vi "Test-Operator-Elevator.vi"() -> ()   [LabVIEW 2014, in "Comp Operator.lvlib"]
uses:
  Comp Operator.lvlib
  Robot Actor Framework/Trace/Trace Controller Class/Config.ctl
  Comp Motors with Encoders/Comp Motors with Encoders Class/Motor Controller Config.ctl
  Robot/Motor with Encoders/Motors with Encoders Class/Motors with Encoders Config.ctl
  Comp Motors with Encoders/Comp Motors with Encoders Class/Encoder Config.ctl
  Robot/Forward Drive/Forward Drive Class/Forward Drive Config.ctl
  Robot/Motor with Encoders/Motors with Encoders Class/Motors with Encoders.lvclass
  Comp Drive/Comp Driver Class/Comp Driver Tuning.ctl
  Robot/Driver/Driver Class/Driver Config.ctl
  Robot/Joystick/Joystick Class/Joystick.lvclass
  <vilib>/ActorFramework/Message Enqueuer/Message Enqueuer.lvclass
  Comp Xbox One Controller/Comp XBox One Controller Class/Comp X1 Config.ctl
  <vilib>/Rock Robotics/WPI/Joystick/WPI_JoystickDeviceEnum.ctl
  Robot/Joystick/Joystick Class/Axis State.ctl
  Robot/Joystick/Joystick Class/Button State.ctl
  Comp Trace Controller/Comp Trace Controller Class/Comp Trace Controller.lvclass
  Comp Pressure/Comp Pressure Class/Comp Pressure.lvclass
  Robot/Forward Drive/Forward Drive Class/Forward Drive.lvclass
  Comp Motors with Encoders/Comp Motors with Encoders Class/Comp Motors with Encoders.lvclass
  Comp Drive/Comp Driver Class/Comp Driver.lvclass
  Comp Xbox One Controller/Comp XBox One Controller Class/Comp XBox One Controller.lvclass
  Comp Xbox One Controller/Comp XBox One Controller Class/Comp XBox One Controller.lvclass/Comp XBox One Controller.ctl
  <vilib>/Rock Robotics/WPI/DriverStation/WPI_DriverStationRobotMode2.ctl
  Robot/Joystick/Joystick Class/Joystick State.ctl
  Robot/Driver/Driver Messages/Drive Forward Drive Msg/Drive Forward Drive Msg.lvclass/Drive Forward Drive Msg.ctl
  <vilib>/ActorFramework/Message Enqueuer/Message Enqueuer.lvclass/Message Enqueuer.ctl
  <vilib>/ActorFramework/Message Enqueuer/Enqueue.vi
  <vilib>/ActorFramework/Message Priority Queue/Priority Enqueue.vi
  Robot/Driver/Driver Messages/Drive Forward Drive Msg/Drive Forward Drive Msg.lvclass
  <vilib>/ActorFramework/Stop Msg/Stop Msg.lvclass
  <vilib>/ActorFramework/Actor/Actor.lvclass
  Robot Actor Framework/Trace/Trace Controller Class/Trace Controller.lvclass
  Robot/Driver/Driver Class/Driver.lvclass
panel:
  in  "Left Back":T1
  in  "Left Right":T1
  in  "Driver - X1 Config":T3={"Joystick USB"=enum."USB 0", "Deadband"=0.05}
  in  "Driver Config":T5={"Joystick"=refnum, "Forward Drive"=refnum, "Sideways Drive"=refnum, "Percent Forward"=1.0, "Percent Sideways"=1.0}
  in  "Comp Driver Tuning":T6={"Control Update Throttle"=75}
  in  "Test Loop":u32=50
  in  "Right Encoder Config":T7={"P"=1.0, "D"=0.0, "F"=0.01, "I"=0.01, "Reverse Feedback Sensor"=TRUE, "Encoder Codes Per Rev"=256}
  in  "Right Slaves":T8[](array[typedef])=[{"Device Number"=5, "Invert Motor"=FALSE}]
  in  "Right Master":T8={"Device Number"=4, "Invert Motor"=TRUE}
  in  "Forward Drive Config":T9={"Left Motors with Encoders"=refnum, "Right Motors with Encoders"=refnum, "Encoder Control"=TRUE}
  in  "Left Encoder Config":T7={"P"=1.0, "D"=0.0, "F"=0.01, "I"=0.01, "Reverse Feedback Sensor"=TRUE, "Encoder Codes Per Rev"=256}
  out "Enable Tele":bool caption="Enabled Teleop"
  in  "Stop Test Loop 1":bool=TRUE
  in  "Finish Test":bool=TRUE
  in  "Start Test":bool=TRUE
  in  "Motors with Encoder Config":T10={"Counts  Per Revolution"=256, "Invert Encoder Direction"=FALSE, "Diameter of Revolution"=6.0, "Max RPM"=1900.0, "Encoder Control"=TRUE}
  in  "Left Slave Motor Controller Configs":T8[](array[typedef])=[{"Device Number"=10, "Invert Motor"=FALSE}]
  in  "left Master Motor Controller Config":T8={"Device Number"=9, "Invert Motor"=FALSE}
  in  "Config":T11={"Folder Pattern"="/media/sd%s1", "Starting Letter Position"=1, "Min Free Space (MB)"=50.0, "Max Folders to Check"=10, "Trace Level"=enum."Debug"} {"Min Free Space (MB)" format="%#_13g"}
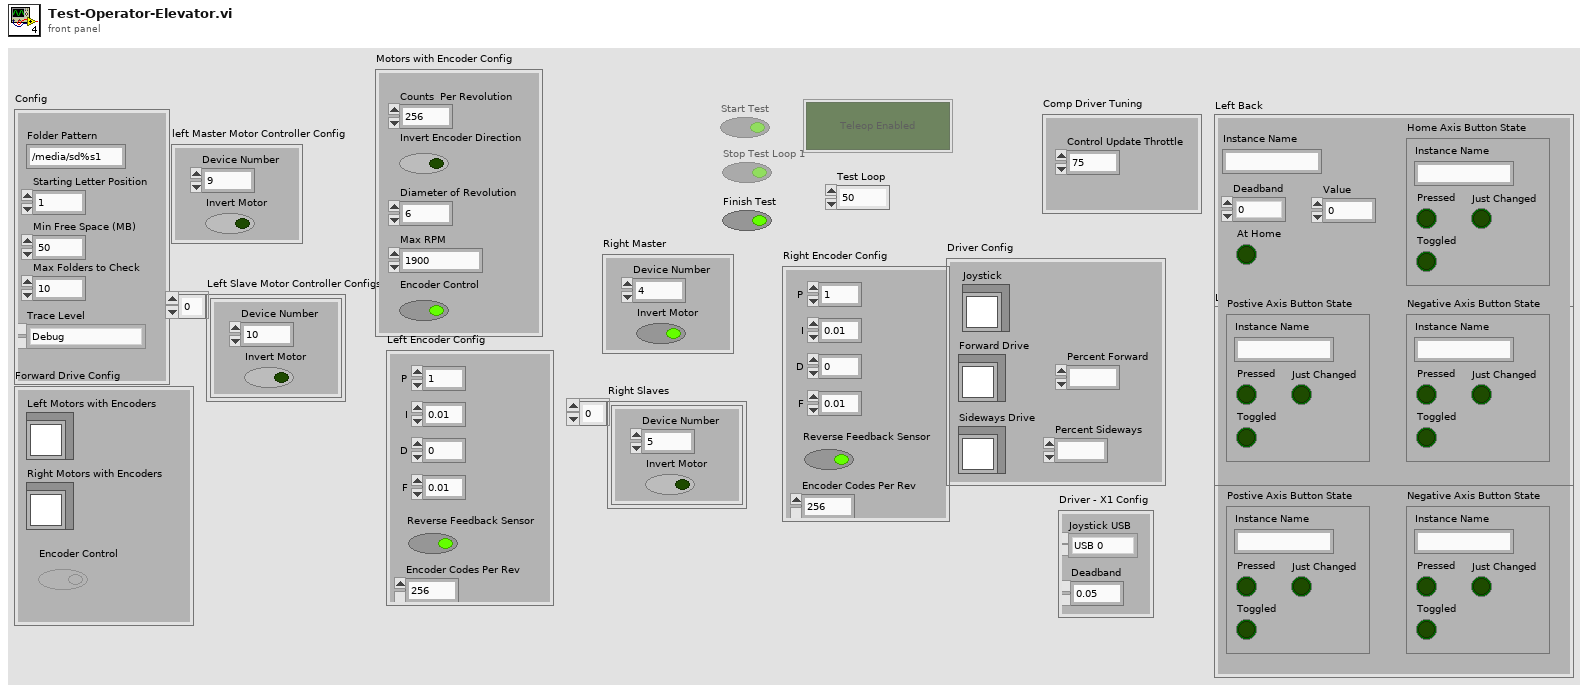
[diagram p1: front panel]
types:
  T1 = typedef "Joystick.lvlib/Joystick.lvclass/Axis State.ctl" = cluster{"Instance Name":string, "Deadband":dbl, "Value":dbl, "At Home":bool, "Postive Axis Button State":T2, "Negative Axis Button State":T2, "Home Axis Button State":T2}
  T2 = typedef "Joystick.lvlib/Joystick.lvclass/Button State.ctl" = cluster{"Pressed":bool, "Instance Name":string, "Toggled":bool, "Just Changed":bool}
  T3 = typedef "Comp XBox One Controller.lvlib/Comp XBox One Controller.lvclass/Comp X1 Config.ctl" = cluster{"Joystick USB":T4, "Deadband":dbl}
  T4 = typedef "WPI_JoystickDeviceEnum.ctl" = enum16{"USB 0", "USB 1", "USB 2", "USB 3", "USB 4", "USB 5"}
  T5 = typedef "Driver.lvlib/Driver.lvclass/Driver Config.ctl" = cluster{"Joystick":refnum<class "Joystick.lvclass">, "Forward Drive":refnum<class "Message Enqueuer.lvclass">, "Sideways Drive":refnum<class "Message Enqueuer.lvclass">, "Percent Forward":dbl, "Percent Sideways":dbl}
  T6 = typedef "Comp Driver.lvlib/Comp Driver.lvclass/Comp Driver Tuning.ctl" = cluster{"Control Update Throttle":u32}
  T7 = typedef "Comp Motors with Encoders.lvlib/Comp Motors with Encoders.lvclass/Encoder Config.ctl" = cluster{"P":dbl, "D":dbl, "F":dbl, "I":dbl, "Reverse Feedback Sensor":bool, "Encoder Codes Per Rev":u16}
  T8 = typedef "Comp Motors with Encoders.lvlib/Comp Motors with Encoders.lvclass/Motor Controller Config.ctl" = cluster{"Device Number":u8, "Invert Motor":bool}
  T9 = typedef "Forward Drive.lvlib/Forward Drive.lvclass/Forward Drive Config.ctl" = cluster{"Left Motors with Encoders":refnum<class "Motors with Encoders.lvclass">, "Right Motors with Encoders":refnum<class "Motors with Encoders.lvclass">, "Encoder Control":bool}
  T10 = typedef "Motors with Encoders.lvlib/Motors with Encoders.lvclass/Motors with Encoders Config.ctl" = cluster{"Counts  Per Revolution":u32, "Invert Encoder Direction":bool, "Diameter of Revolution":dbl, "Max RPM":dbl, "Encoder Control":bool}
  T11 = typedef "Robot Actor Framework.lvlib/Trace.lvlib/Trace Controller.lvclass/Config.ctl" = cluster{"Folder Pattern":string, "Starting Letter Position":i32, "Min Free Space (MB)":dbl, "Max Folders to Check":u32, "Trace Level":enum16{"Critical", "Error", "Warning", "Informational", "Debug"}}
  T12 = enum16{"Critical", "Error", "Warning", "Informational", "Debug"}
  T13 = enum8{"Enabled", "Disabled", "Disabled and Grayed Out"}
  T14 = typedef "WPI_DriverStationRobotMode2.ctl" = enum16{"Autonomous Disabled", "Autonomous Enabled", "Teleop Disabled", "Teleop Enabled", "Disconnected", "Finish", "Test Disabled", "Test Enabled", "Emergency Stopped"}
  T15 = typedef "Joystick.lvlib/Joystick.lvclass/Joystick State.ctl" = cluster{"Buttons":T2[], "Axis":T1[]}
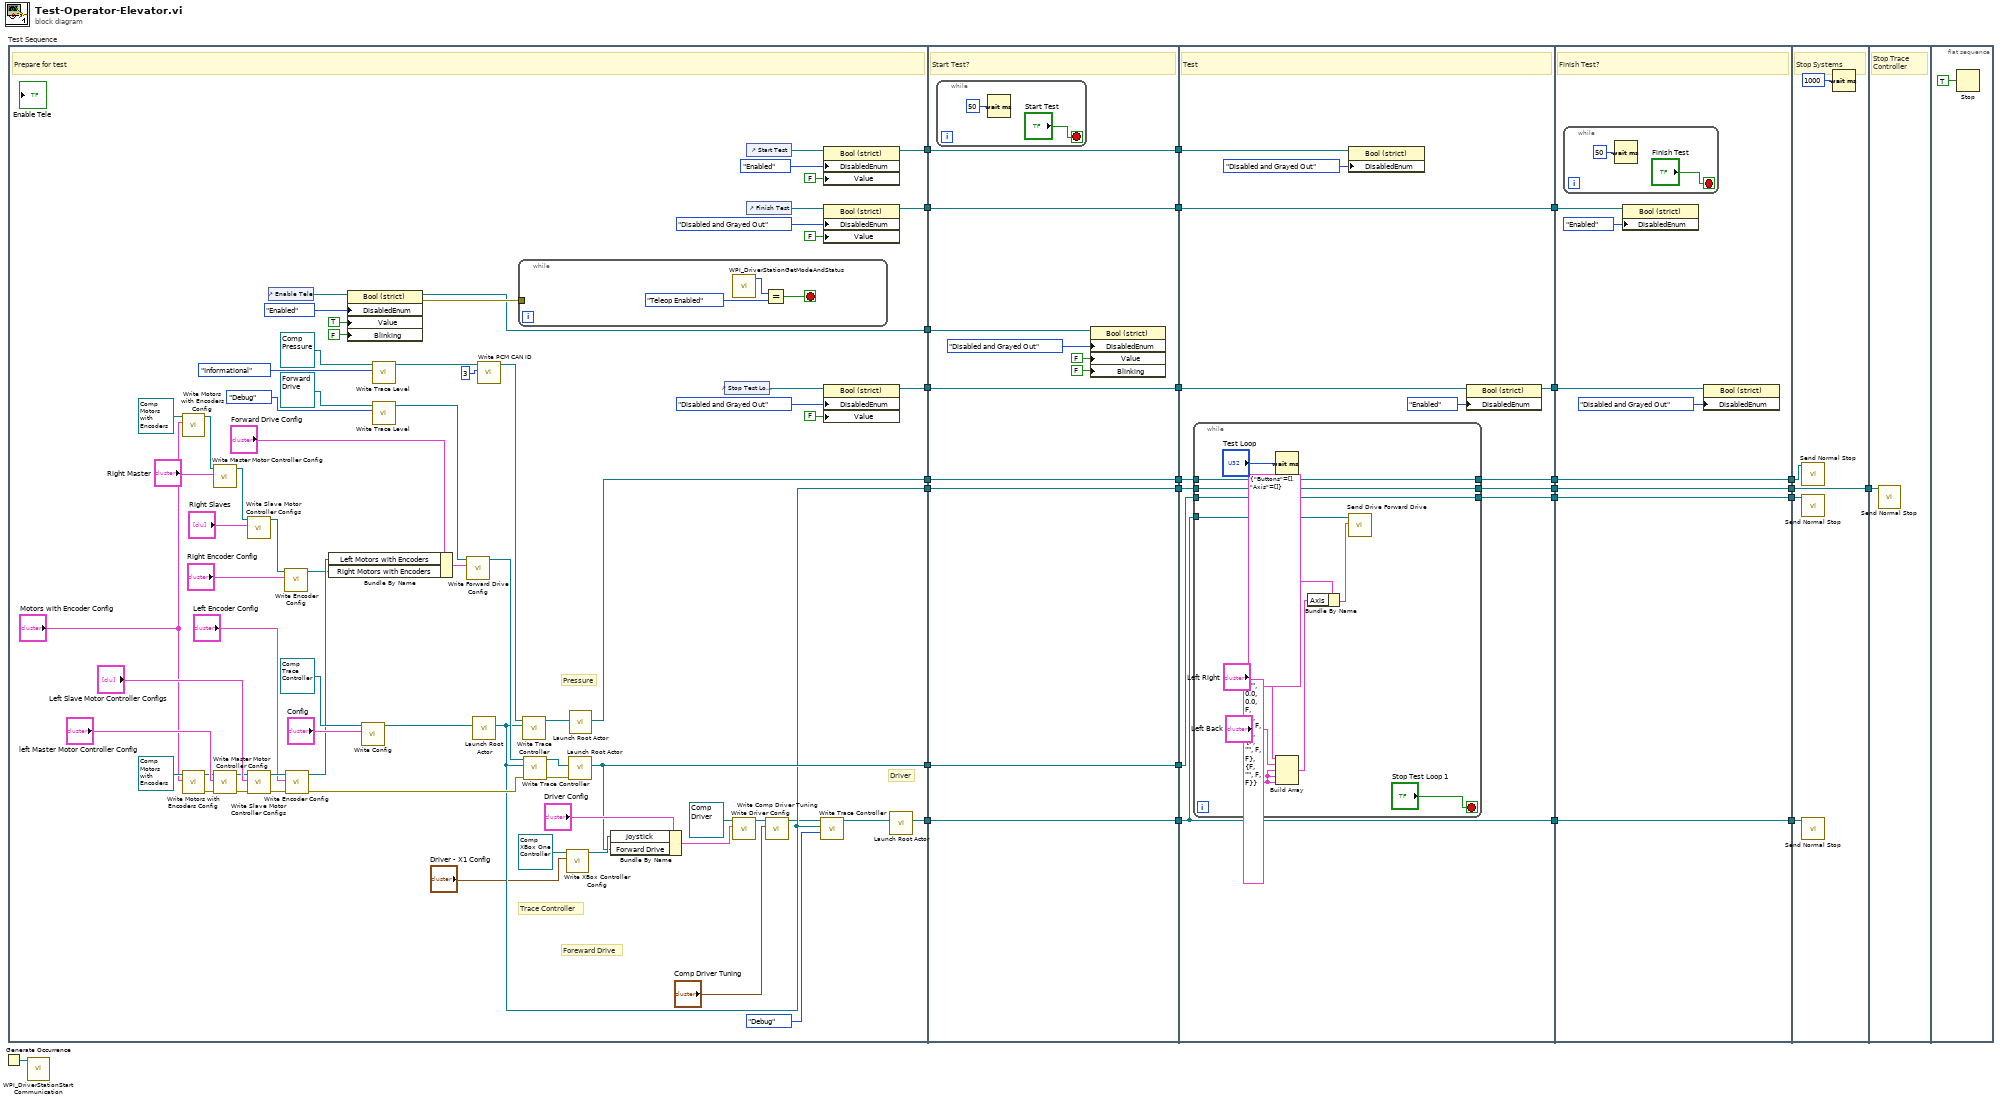
[diagram p0: block diagram]
diagram:
  n1 = Generate Occurrence() -> (w27:refnum<k4>)
  n2 = flat-sequence "Test Sequence" {
    tunnel: [w34] -> w16
    tunnel: [w82] -> w15
    tunnel: [w33] -> w14
    tunnel: [w72] -> w13
    tunnel: [w71] -> w11
    tunnel: [w70] -> w6
    tunnel: [w64] -> w5
    tunnel: [w30] -> w3
    tunnel: [w112] -> w19
    tunnel: [w111] -> w18
    tunnel: [w110] -> w17
    tunnel: w16 -> [w112]
    tunnel: w15 -> [w111]
    tunnel: w14 -> [w110]
    tunnel: w13 -> [w109]
    tunnel: [w109] -> w12
    tunnel: w11 -> [w108]
    tunnel: [w108] -> w10
    tunnel: [w107] -> w7
    tunnel: w6 -> [w107]
    tunnel: w5 -> [w106]
    tunnel: [w102] -> w4
    tunnel: w3 -> [w102]
    tunnel: [w122] -> w22
    tunnel: [w124] -> w21
    tunnel: [w123] -> w20
    tunnel: w19 -> [w127]
    tunnel: w18 -> [w125]
    tunnel: w17 -> [w126]
    tunnel: w12 -> [w121]
    tunnel: w10 -> [w119]
    tunnel: [w117] -> w9
    tunnel: [w116] -> w8
    tunnel: w7 -> [w116]
    tunnel: w4 -> [w115]
    tunnel: [w115] -> w1
    tunnel: [w147] -> w25
    tunnel: [w146] -> w24
    tunnel: [w145] -> w23
    tunnel: w22 -> [w147]
    tunnel: w21 -> [w146]
    tunnel: w20 -> [w145]
    tunnel: w9 -> [w144]
    tunnel: w8 -> [w141]
    tunnel: [w140] -> w2
    tunnel: w1 -> [w140]
    tunnel: [w154] -> w26
    tunnel: w25 -> [w154]
    tunnel: w24 -> [w153]
    tunnel: w23 -> [w151]
    tunnel: w2 -> [w150]
    tunnel: w26 -> [w155]
    frame #0 {
      # "Driver"
      # "Trace Controller"
      # "Pressure"
      # "Foreward Drive"
      # "Prepare for test"
      n3 = call-dynamic "Write Motors with Encoders Config.vi"("Motors with Encoders Config"="Motors with Encoder Config", "Motors with Encoders in"=refnum<class "Comp Motors with Encoders.lvclass"> refnum ("Comp Motors with Encoders.lvlib:Comp Motors with Encoders.lvclass")) -> ("Motors with Encoders out"=w50:refnum<class "Comp Motors with Encoders.lvclass">)  [unwired: 8 in, 1 out]
      n4 = call-dynamic "Write Motors with Encoders Config.vi"("Motors with Encoders Config"="Motors with Encoder Config", "Motors with Encoders in"=refnum<class "Comp Motors with Encoders.lvclass"> refnum ("Comp Motors with Encoders.lvlib:Comp Motors with Encoders.lvclass")) -> ("error out"=w89:errorcluster, "Motors with Encoders out"=w52:refnum<class "Comp Motors with Encoders.lvclass">)  [unwired: 8 in]
      n5 = call-dynamic "Write Master Motor Controller Config.vi"("Master Motor Controller Config"="Right Master", "Comp Motors with Encoders in"=w50) -> ("Comp Motors with Encoders out"=w49:refnum<class "Comp Motors with Encoders.lvclass">)  [unwired: 8 in, 1 out]
      n6 = call-dynamic "Write Master Motor Controller Config.vi"("error in (no error)"=w89, "Master Motor Controller Config"="left Master Motor Controller Config", "Comp Motors with Encoders in"=w52) -> ("error out"=w90:errorcluster, "Comp Motors with Encoders out"=w86:refnum<class "Comp Motors with Encoders.lvclass">)  [unwired: 7 in]
      n7 = call-dynamic "Write Slave Motor Controller Configs.vi"("Slave Motor Controller Configs"="Right Slaves", "Comp Motors with Encoders in"=w49) -> ("Comp Motors with Encoders out"=w48:refnum<class "Comp Motors with Encoders.lvclass">)  [unwired: 8 in, 1 out]
      n8 = call-dynamic "Write Slave Motor Controller Configs.vi"("error in (no error)"=w90, "Slave Motor Controller Configs"="Left Slave Motor Controller Configs", "Comp Motors with Encoders in"=w86) -> ("error out"=w62:errorcluster, "Comp Motors with Encoders out"=w63:refnum<class "Comp Motors with Encoders.lvclass">)  [unwired: 7 in]
      n9 = control-ref of="Enable Tele"() -> (w69:refnum<vi>)
      n10 = call-dynamic "Write Encoder Config.vi"("Encoder Config"="Right Encoder Config", "Comp Motors with Encoders in"=w48) -> ("Comp Motors with Encoders out"=w47:refnum<class "Comp Motors with Encoders.lvclass">)  [unwired: 8 in, 1 out]
      n11 = call-dynamic "Write Encoder Config.vi"("error in (no error)"=w62, "Encoder Config"="Left Encoder Config", "Comp Motors with Encoders in"=w63) -> ("error out"=w61:errorcluster, "Comp Motors with Encoders out"=w58:refnum<class "Comp Motors with Encoders.lvclass">)  [unwired: 7 in]
      n12 = Bundle By Name(cluster="Forward Drive Config", "Left Motors with Encoders"=w58, "Right Motors with Encoders"=w47) -> (w59:T9)
      n13 = property class="Bool (strict)"(reference=w69, "DisabledEnum"=T13."Enabled" ("Disabled"), "Value"=TRUE, "Blinking"=FALSE) -> (reference out=w64:refnum<vi>, error out=w66:errorcluster)  [unwired: 1 in]
      n14 = call-dynamic "Write Config.vi"("Config"="Config", "Trace Controller in"=refnum<class "Comp Trace Controller.lvclass"> refnum ("Comp Trace Controller.lvlib:Comp Trace Controller.lvclass")) -> ("Trace Controller out"=w85:refnum<class "Comp Trace Controller.lvclass">)  [unwired: 8 in, 1 out]
      n15 = call-dynamic "Write Trace Level.vi"("Trace Level"=T12."Informational", "System Actor in"=refnum<class "Comp Pressure.lvclass"> refnum ("Comp Pressure.lvlib:Comp Pressure.lvclass")) -> ("System Actor out"=w95:refnum<class "Comp Pressure.lvclass">)  [unwired: 8 in, 1 out]
      n16 = call-dynamic "Write Trace Level.vi"("Trace Level"=T12."Debug", "System Actor in"=refnum<class "Forward Drive.lvclass"> refnum ("Forward Drive.lvlib:Forward Drive.lvclass")) -> ("System Actor out"=w55:refnum<class "Forward Drive.lvclass">)  [unwired: 8 in, 1 out]
      n17 = call-dynamic "Write Forward Drive Config.vi"("Forward Drive Config"=w59, "Forward Drive in"=w55) -> ("Forward Drive out"=w57:refnum<class "Forward Drive.lvclass">)  [unwired: 8 in, 1 out]
      n18 = call <vilib>:"Launch Root Actor.vi"("Actor"=w85) -> ("Actor's Enqueuer"=w33:refnum<class "Message Enqueuer.lvclass">)  [unwired: 9 in, 1 out]
      n19 = call-dynamic "Write PCM CAN ID.vi"("PCM CAN ID"=u8 3, "Comp Pressure in"=w95) -> ("Comp Pressure out"=w97:refnum<class "Comp Pressure.lvclass">)  [unwired: 8 in, 1 out]
      n20 = while {
        tunnel: w66 -> [_]
        stop <- w99 stop-if-true
        n21 = call <vilib>:"WPI_DriverStationGetModeAndStatus.vi"() -> ("Robot Mode"=w101:T14)  [unwired: 10 in, 1 out]
        n22 = Equal?(x=w101, y=WPI_DriverStationRobotMode2."Teleop Enabled") -> (x = y?=w99:bool)
      }
      n23 = call-dynamic "Write Trace Controller.vi"("Trace Controller"=w33, "System Actor in"=w97) -> ("System Actor out"=w98:refnum<class "Comp Pressure.lvclass">)  [unwired: 8 in, 1 out]
      n24 = call-dynamic "Write Trace Controller.vi"("error in (no error)"=w61, "Trace Controller"=w33, "System Actor in"=w57) -> ("error out"=w92:errorcluster, "System Actor out"=w91:refnum<class "Forward Drive.lvclass">)  [unwired: 7 in]
      n25 = call "Write XBox Controller Config.vi"("XBox One Controller Config"="Driver - X1 Config", "Comp XBox One Controller in"=refnum<class "Comp XBox One Controller.lvclass"> refnum ("Comp XBox One Controller.lvlib:Comp XBox One Controller.lvclass")) -> ("Comp XBox One Controller out"=w35:refnum<class "Comp XBox One Controller.lvclass">)  [unwired: 8 in, 1 out]
      n26 = call <vilib>:"Launch Root Actor.vi"("error in (no error)"=w92, "Actor"=w91) -> ("Actor's Enqueuer"=w34:refnum<class "Message Enqueuer.lvclass">)  [unwired: 8 in, 1 out]
      n27 = call <vilib>:"Launch Root Actor.vi"("Actor"=w98) -> ("Actor's Enqueuer"=w82:refnum<class "Message Enqueuer.lvclass">)  [unwired: 9 in, 1 out]
      n28 = Bundle By Name(cluster="Driver Config", "Joystick"=w35, "Forward Drive"=w34) -> (w36:T5)
      n29 = control-ref of="Stop Test Loop 1"() -> (w76:refnum<vi>)
      n30 = call-dynamic "Write Driver Config.vi"("Driver Config"=w36, "Driver in"=refnum<class "Comp Driver.lvclass"> refnum ("Comp Driver.lvlib:Comp Driver.lvclass")) -> ("Driver out"=w37:refnum<class "Comp Driver.lvclass">)  [unwired: 8 in, 1 out]
      n31 = control-ref of="Start Test"() -> (w81:refnum<vi>)
      n32 = control-ref of="Finish Test"() -> (w75:refnum<vi>)
      n33 = call-dynamic "Write Comp Driver Tuning.vi"("Comp Driver Tuning"="Comp Driver Tuning", "Comp Driver in"=w37) -> ("Comp Driver out"=w28:refnum<class "Comp Driver.lvclass">)  [unwired: 8 in, 1 out]
      n34 = call-dynamic "Write Trace Controller.vi"("Trace Level"=T12."Debug", "Trace Controller"=w33, "System Actor in"=w28) -> ("System Actor out"=w32:refnum<class "Comp Driver.lvclass">)  [unwired: 7 in, 1 out]
      n35 = property class="Bool (strict)"(reference=w81, "DisabledEnum"=T13."Enabled" ("Disabled"), "Value"=FALSE) -> (reference out=w72:refnum<vi>)  [unwired: 1 in, 1 out]
      n36 = property class="Bool (strict)"(reference=w75, "DisabledEnum"=T13."Disabled and Grayed Out" ("Disabled"), "Value"=FALSE) -> (reference out=w70:refnum<vi>)  [unwired: 1 in, 1 out]
      n37 = property class="Bool (strict)"(reference=w76, "DisabledEnum"=T13."Disabled and Grayed Out" ("Disabled"), "Value"=FALSE) -> (reference out=w71:refnum<vi>)  [unwired: 1 in, 1 out]
      n38 = call <vilib>:"Launch Root Actor.vi"("Actor"=w32) -> ("Actor's Enqueuer"=w30:refnum<class "Message Enqueuer.lvclass">)  [unwired: 9 in, 1 out]
    }
    frame #1 {
      # "Start Test?"
      n39 = while {
        stop <- "Start Test" stop-if-true
        n40 = Wait (ms)(milliseconds to wait=u32 50) -> ()  [unwired: 1 out]
      }
      n41 = property class="Bool (strict)"(reference=w106, "DisabledEnum"=T13."Disabled and Grayed Out" ("Disabled"), "Value"=FALSE, "Blinking"=FALSE) -> ()  [unwired: 1 in, 2 out]
    }
    frame #2 {
      # "Test"
      n42 = while {
        tunnel: w126 -> [w139]
        tunnel: [w139] -> w122
        tunnel: w127 -> [w136]
        tunnel: [w136] -> w124
        tunnel: w125 -> [w138]
        tunnel: [w138] -> w123
        tunnel: w115 -> [w135]
        stop <- "Stop Test Loop 1" stop-if-true
        w134 = T1 {"Instance Name"="", "Deadband"=0.0, "Value"=0.0, "At Home"=FALSE, "Postive Axis Button State"={"Pressed"=FALSE, "Instance Name"="", "Toggled"=FALSE, "Just Changed"=FALSE}, "Negative Axis Button State"={"Pressed"=FALSE, "Instance Name"="", "Toggled"=FALSE, "Just Changed"=FALSE}, "Home Axis Button State"={"Pressed"=FALSE, "Instance Name"="", "Toggled"=FALSE, "Just Changed"=FALSE}} ("Axis State")
        n43 = Wait (ms)(milliseconds to wait="Test Loop") -> ()  [unwired: 1 out]
        n44 = Build Array("Left Right", "Left Back", w134, w134, w134) -> (w131:T1[])
        n45 = Bundle By Name(cluster=T15 {"Buttons"=[], "Axis"=[]} ("Joystick State"), "Axis"=w131) -> (w132:T15)
        n46 = call "Send Drive Forward Drive.vi"("Joystick State"=w132, "Message Enqueuer"=w135) -> ()  [unwired: 8 in, 2 out]
      }
      n47 = property class="Bool (strict)"(reference=w121, "DisabledEnum"=T13."Disabled and Grayed Out" ("Disabled")) -> ()  [unwired: 1 in, 2 out]
      n48 = property class="Bool (strict)"(reference=w119, "DisabledEnum"=T13."Enabled" ("Disabled")) -> (reference out=w117:refnum<vi>)  [unwired: 1 in, 1 out]
    }
    frame #3 {
      # "Finish Test?"
      n49 = while {
        stop <- "Finish Test" stop-if-true
        n50 = Wait (ms)(milliseconds to wait=u32 50) -> ()  [unwired: 1 out]
      }
      n51 = property class="Bool (strict)"(reference=w141, "DisabledEnum"=T13."Enabled" ("Disabled")) -> ()  [unwired: 1 in, 2 out]
      n52 = property class="Bool (strict)"(reference=w144, "DisabledEnum"=T13."Disabled and Grayed Out" ("Disabled")) -> ()  [unwired: 1 in, 2 out]
    }
    frame #4 {
      # "Stop Systems"
      n53 = call <vilib>:"Send Normal Stop.vi"("Message Enqueuer"=w151) -> ()  [unwired: 10 in, 1 out]
      n54 = call <vilib>:"Send Normal Stop.vi"("Message Enqueuer"=w153) -> ()  [unwired: 10 in, 1 out]
      n55 = call <vilib>:"Send Normal Stop.vi"("Message Enqueuer"=w150) -> ()  [unwired: 10 in, 1 out]
      n56 = Wait (ms)(milliseconds to wait=u32 1000) -> ()  [unwired: 1 out]
    }
    frame #5 {
      # "Stop Trace Controller"
      n57 = call <vilib>:"Send Normal Stop.vi"("Message Enqueuer"=w155) -> ()  [unwired: 10 in, 1 out]
    }
    frame #6 {
      n58 = Stop(stop? (T)=TRUE) -> ()
    }
  }
  n59 = call <vilib>:"WPI_DriverStationStart Communication.vi"("occurrence"=w27) -> ()  [unwired: 1 in, 10 out]
